vi "subProcessClass.vi"(8 "error in (no error)":errorcluster, 9 "Blacklist Class":T1, 10 "VI Refnum":refnum<vi>, 11 "CLI":refnum<class "CLI.lvclass">) -> (0 "error out":errorcluster, 1 "Reject?":bool, 2 "dup VI Refnum":refnum<vi>, 3 "CLI out":refnum<class "CLI.lvclass">)   [LabVIEW 2014, in "lvbuildsecurity.lvlib"]
uses:
  lvbuildsecurity.lvlib
  ctlBlacklistClass.ctl
  <vilib>/Wiresmith Technology/LabVIEW CLI/CLI Class/CLI.lvclass
  classes/Blacklist.lvclass
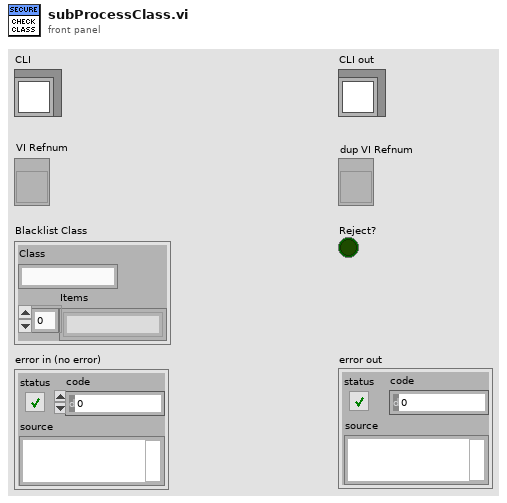
[diagram p1: front panel]
types:
  T1 = typedef "lvbuildsecurity.lvlib/ctlBlacklistClass.ctl" = cluster{"Class":string, "Items":string[]}
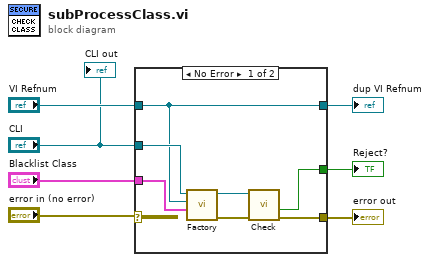
[diagram p0: block diagram]
diagram:
  n1 = case shown="No Error" "error in (no error)" {
    selector: "error in (no error)" -> [_ w16]
    tunnel: "Blacklist Class" -> [w9 _]
    tunnel: [w12 w16] -> w4
    tunnel: "VI Refnum" -> [w8 w15]
    tunnel: [w8 w15] -> w2
    tunnel: [w11 _] -> w3
    tunnel: "CLI" -> [w10 _]
    frame No Error {
      n2 = call "Factory.vi"("Blacklist Class"=w9, "VI Refnum"=w8, "CLI"=w10) -> ("error out"=w13:errorcluster, "Blacklist out"=w14:refnum<class "Blacklist.lvclass">)  [unwired: 7 in]
      n3 = call "Check.vi"("error in (no error)"=w13, "Blacklist in"=w14) -> ("error out"=w12:errorcluster, "Reject?"=w11:bool)  [unwired: 7 in, 1 out]
    }
    frame Error {
    }
  }
  "error out" <- w4
  "Reject?" <- w3
  "dup VI Refnum" <- w2
  "CLI out" <- "CLI"
